vi "daq.io Embedded Machine Example Token.vi"(8 "error in":errorcluster) -> (0 "error out":errorcluster)   [LabVIEW 2013, in "daqio minimal.lvlib"]
doc: "This interactive example demonstrates how an NI Embedded device can used for continuous monitoring with daq.io. Tags and Events in this example are written on user demand but could also be triggered by monitored values. \n\nTo get started, <b>drag this example onto a Real-Time target in the Project Explorer, enter a valid Token in the block diagram</b> and run it interactively. You can also build an Executable and run it upon startup. To generate a Token, log in to your account on daq.io and go to your user page (click your user name next to logout button).\n\nThe NI System Configuration API is being used to monitor the status of the Embedded device. Please make sure its libraries are installed on the Embedded Device to get the best experience."
uses:
  daqio minimal.lvlib
  _typedefs/update-button.ctl
  _typedefs/trigger-button.ctl
  _typedefs/exmpl-states.ctl
  _typedefs/connection_FGV_commands.ctl
  _typedefs/daqio-reconnect-status.ctl
  _typedefs/daqio-Buffer-Commands.ctl
  <vilib>/nisyscfg/Close (System).vi
  _subs/daqio_Write_Multiple_single_Timestamp.vi
  <resource>/objmgr/nisysapi.rc
  <vilib>/nisyscfg/nisyscfg.lvlib
panel:
  out "Setpoint":dbl(slide) scale=0.0..150.0
  out "shutdown":bool
  out "Log":string[](array[string])
  in  "Stop":bool
  in  "Fire Event":T1
  in  "Select Event":u16(ring) items=["Safety Hood Status", "Manual Operation", "Shutting Down"]
  out "Time Stamp sent":timestamp
  in  "Event Data":string
  in  "Update Tags":T2
  out "connected":bool
  out "Speed (RPM)":dbl(knob) scale=0.0..2000.0
  out "Temperature Data":dbl(graph)
  out "RAM":dbl(slide) scale=0.0..100.0
  out "CPU":dbl(slide) scale=0.0..100.0
  in  "Value 3":string="1234-abc"
  in  "Value 2":string="XYZ 3000 Plus"
  in  "Tag 3":string="Serial Number"
  in  "Tag 2":string="Type"
  in  "Value 1":string="47.615459, -122.323804"
  in  "Tag 1":string="Location"
  out "Device Key":string
  # "Get your free account at daq.io first: sign up at daq.io."
  # "This Machine"
  # "(autogenerated in this example)"
  # "Please enter your \nToken in the block \ndiagram. Generate \nyour Token online."
  # "Device Tags"
  # "Use device tags to describe \nspecific parameters for each\ndevice. These can include the \nlocation, the serial number or\nother machine or location-\nspecific information. These\nfields are fully user-defined."
  # "Device Events"
  # "Use device events to signal\nany local event to daq.io. These\ncould include mechanical events\n(e.g. \"safety latch released\") or \nany change on the device that\nneeds to be tracked."
  # "Device Live Data Channels"
  # "Use device channels to transfer\ntime series data. All channels \nof the device will be visible in \nthe online data viewer. You \ncan build your own dashboard \nin the webbrowser and link it\nto exisiting channels."
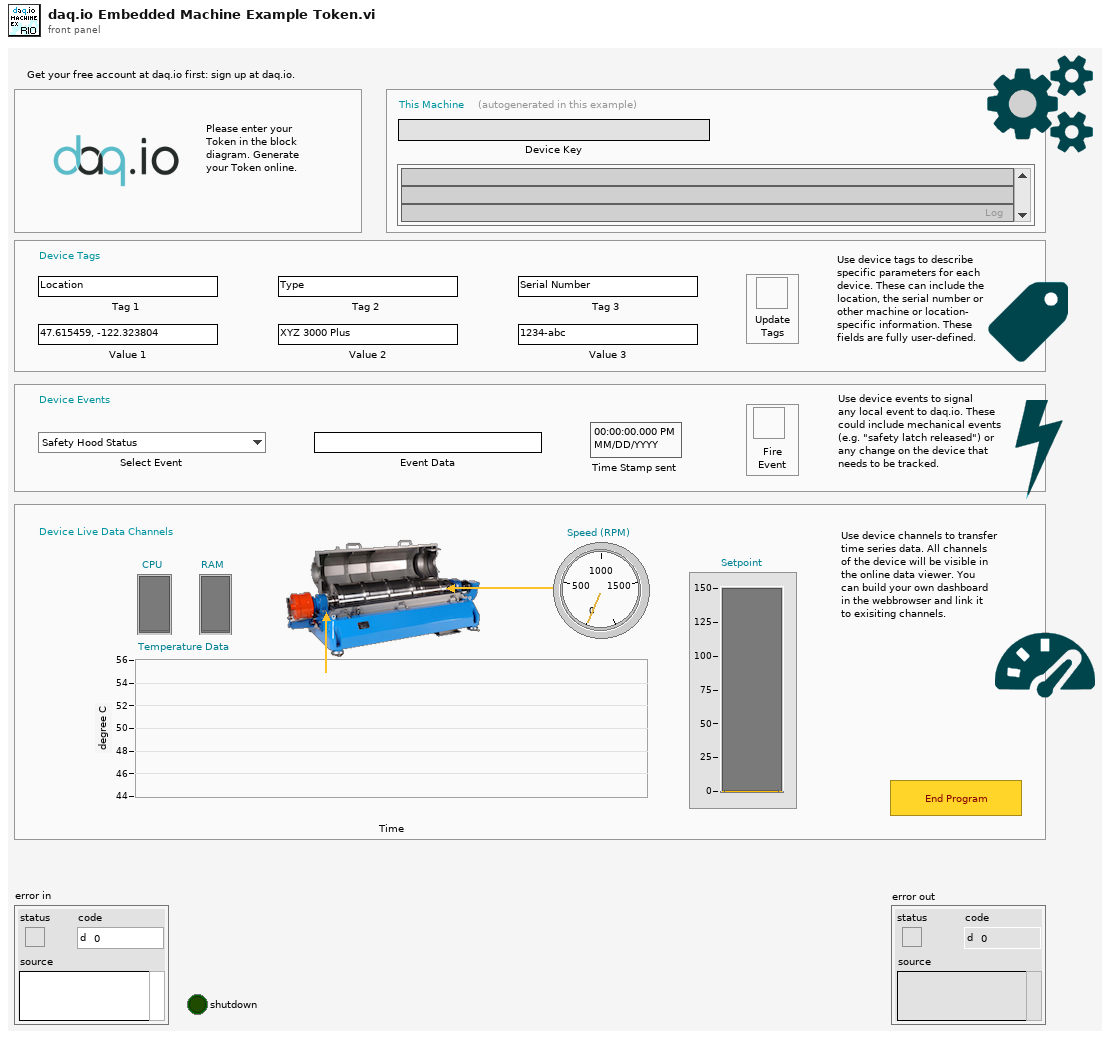
[diagram p1: front panel]
types:
  T1 = typedef "daqio minimal.lvlib/trigger-button.ctl" = bool
  T2 = typedef "daqio minimal.lvlib/update-button.ctl" = bool
  T3 = typedef "daqio minimal.lvlib/exmpl-states.ctl" = enum16{"idle", "time series", "fire events", "update tags", "end program", "create waveform", "create dashboard"}
  T4 = typedef "daqio minimal.lvlib/daqio-Type.ctl" = cluster{"daq.io ref":T5, "daq.io API Base":string, "Device Key":string, "Account ID":string, "online":bool, "SSL":bool}
  T5 = typedef "LabVIEWHTTPClient.lvlib/ClientHandle.ctl" = refnum<k1>
  T6 = typedef "daqio minimal.lvlib/connection_FGV_commands.ctl" = enum16{"Set Conn Stat", "Save Type", "Get Type from File", "Set Type", "Set Buffer", "Get"}
  T7 = typedef "daqio minimal.lvlib/daqio-reconnect-status.ctl" = enum16{"Reconnect success", "Reconnect failed", "Connected", "Offline"}
  T8 = typedef "daqio minimal.lvlib/daqio-Buffer-Commands.ctl" = enum16{"Add to Buffer", "Post from Buffer", "Clear Buffer", "Init"}
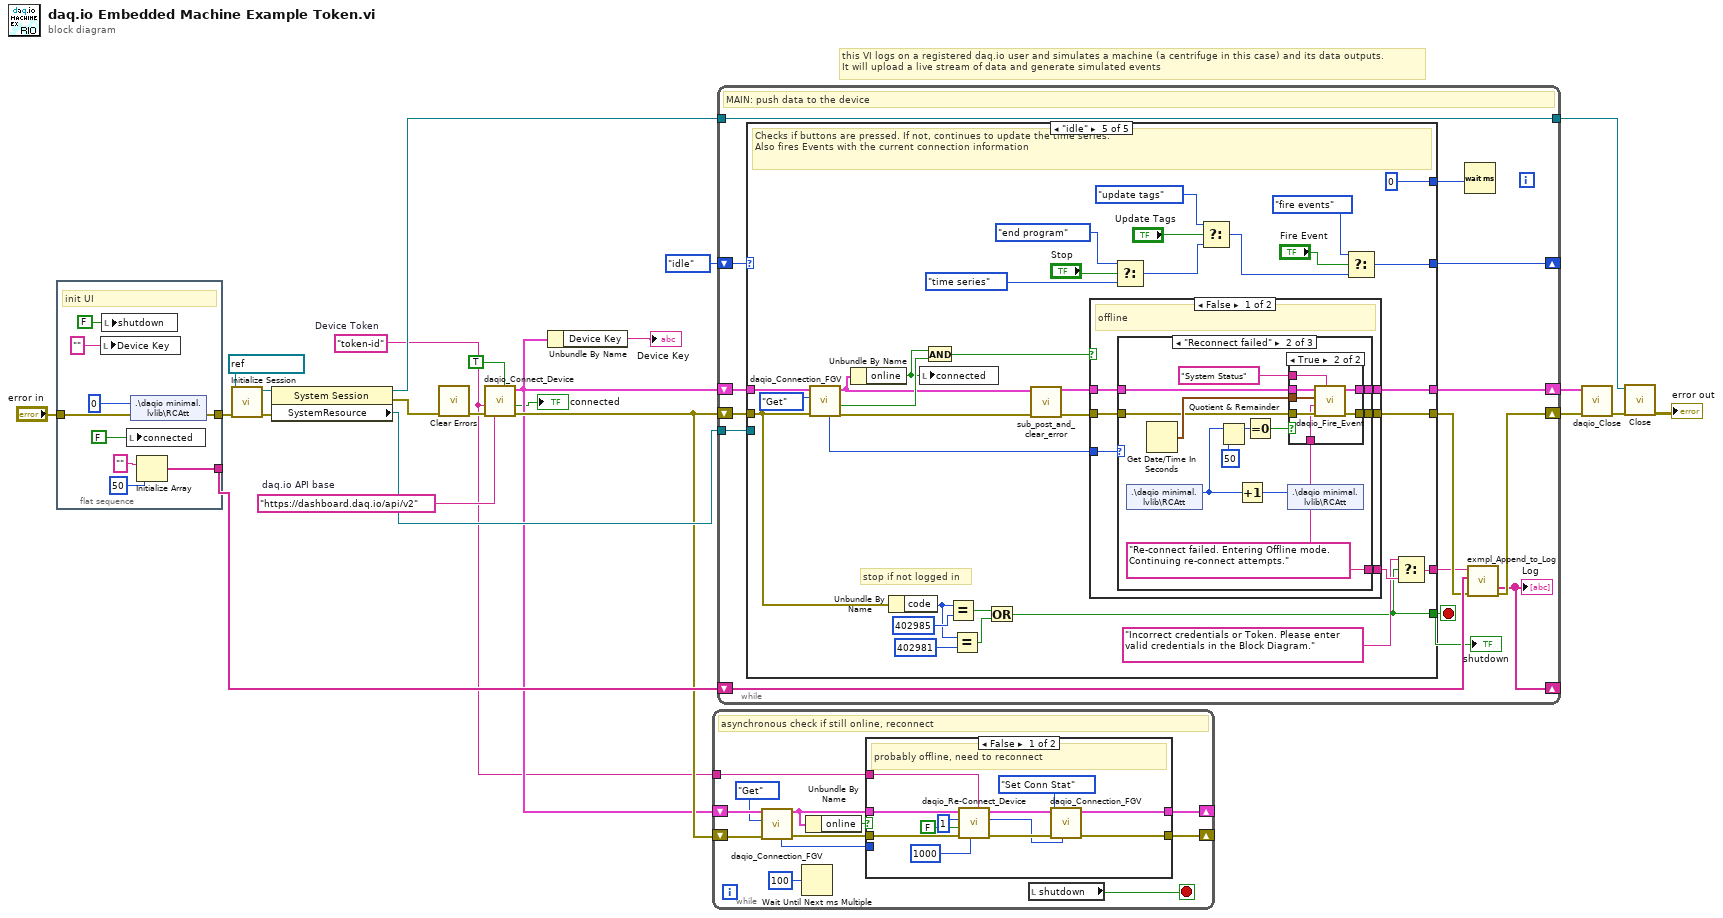
[diagram p0: block diagram]
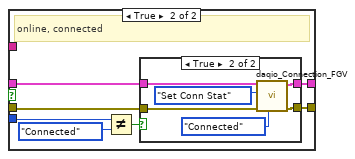
[diagram p2: hidden frame]
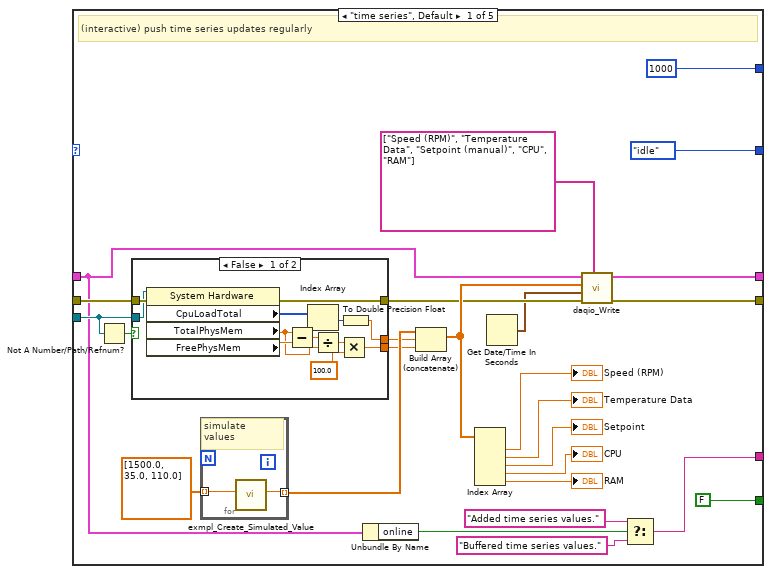
[diagram p4: hidden frame]
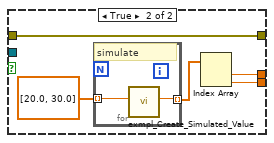
[diagram p5: hidden frame]
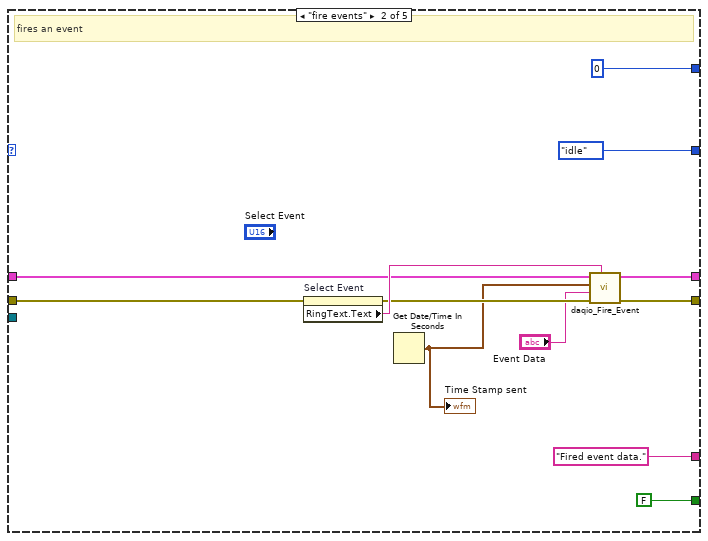
[diagram p6: hidden frame]
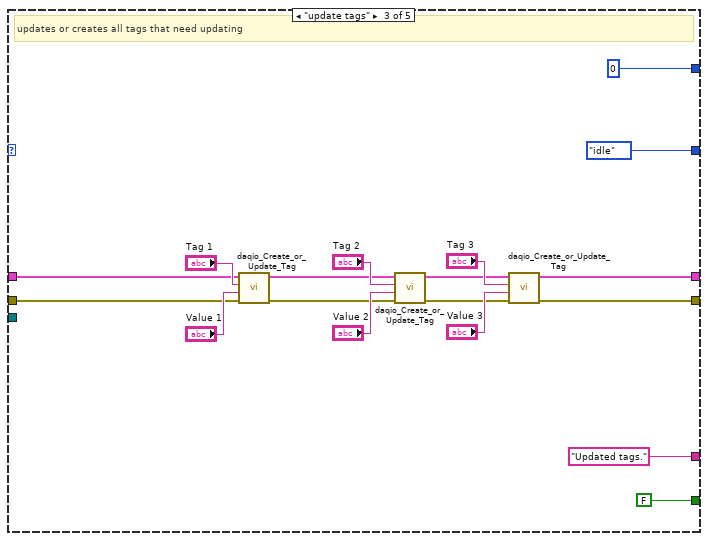
[diagram p7: hidden frame]
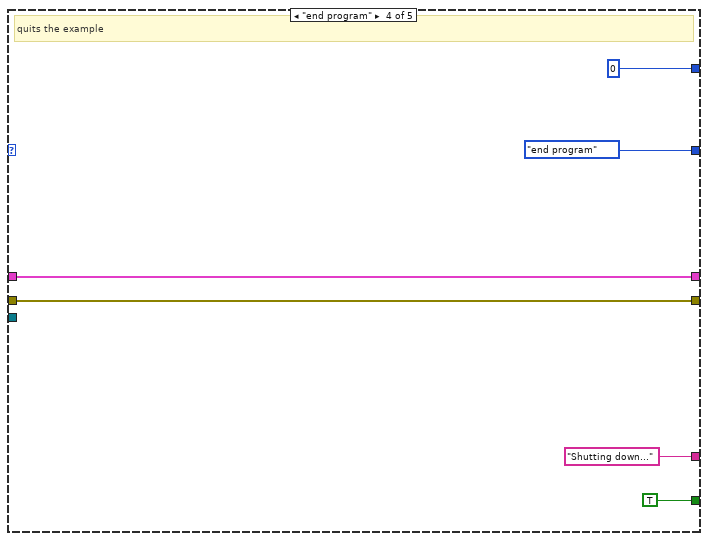
[diagram p8: hidden frame]
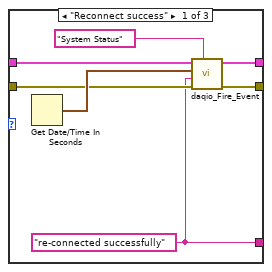
[diagram p9: hidden frame]
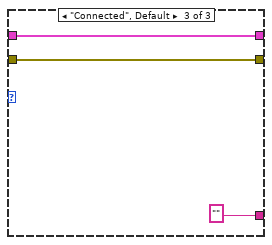
[diagram p11: hidden frame]
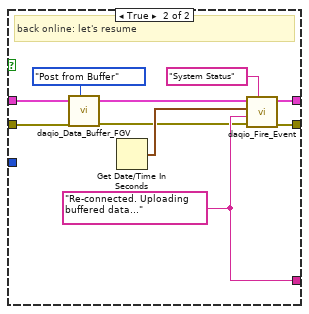
[diagram p12: hidden frame]
diagram:
  w1 = "token-id"  # Device Token
  w20 = "https://dashboard.daq.io/api/v2"  # daq.io API base
  # "this VI logs on a registered daq.io user and simulates a machine (a centrifuge in this case) and its data outputs. \nIt will upload a live stream of data and generate simulated events"
  n1 = flat-sequence {
    tunnel: [w26] -> w18
    tunnel: "error in" -> [w28]
    tunnel: [w29] -> w7
    frame #0 {
      # "init UI"
      n2 = local write "Device Key"("" ("log")) -> ()
      n3 = local write "shutdown"(FALSE ("shutdown")) -> ()
      n4 = local write "connected"(FALSE ("connected to daq.io")) -> ()
      n5 = shared-variable ".\\daqio minimal.lvlib\\RCAtt"(0 ("RCAtt"), error in=w28) -> (error out=w26:errorcluster)
      n6 = Initialize Array("" ("log"), 50 ("dimension size")) -> (w29:string[])
    }
  }
  n7 = call <vilib>:"Initialize Session.vi"("error in (no error)"=w18, "Target (localhost)"=refnum<k21> "localhost" ("Embedded Target (self)")) -> ("error out"=w12:errorcluster, "Session out"=w10:refnum<k21>)  [unwired: 8 in]
  n8 = property class="System Session"(reference=w10, error in=w12) -> (reference out=w9:refnum<k21>, error out=w11:errorcluster, "SystemResource"=w13:refnum<k20>)
  n9 = call <vilib>:"Clear Errors.vi"("error in (no error)"=w11) -> ("error out"=w4:errorcluster)  [unwired: 6 in]
  n10 = call "daqio_Connect_Device.vi"("Use SSL"=TRUE, "daq.io API base"=w20, "error in (no error)"=w4, "Device Token"=w1) -> ("error out"=w6:errorcluster, "connected successfully?"=→"connected":bool, "daq.io type out"=w5:T4)  [unwired: 5 in]
  n11 = Unbundle By Name(w5) -> ("Device Key"=→"Device Key":string)
  n12 = while {
    shift-right: [w37] -> _
    shift-left: w6 -> [w41]
    shift-right: [w38] -> _
    shift-left: w5 -> [w42]
    tunnel: w1 -> [w33]
    stop <- w44 stop-if-true
    # "asynchronous check if still online, reconnect"
    n13 = call "daqio_Connection_FGV.vi"("error in"=w41, "Enum"=connection_FGV_commands."Get", "daq.io type in"=w42) -> ("error out"=w39:errorcluster, "daq.io type out"=w35:T4, "Connection Status out"=w34:T7)  [unwired: 5 in, 1 out]
    n14 = Wait Until Next ms Multiple(millisecond multiple=u32 100) -> ()  [unwired: 1 out]
    n15 = Unbundle By Name(w35) -> ("online"=w36:bool)
    n16 = case shown="False" w36 {
      tunnel: w39 -> [w54 w58]
      tunnel: [w49 w61] -> w38
      tunnel: [w48 w60] -> w37
      tunnel: w35 -> [w47 w59]
      tunnel: w34 -> [_ w63]
      tunnel: w33 -> [w45 _]
      frame False {
        # "probably offline, need to reconnect"
        n17 = call "daqio_Re-Connect_Device.vi"("Token"=w45, "re-connect timeouts"=u32 1000, "error in"=w54, "override any errors"=FALSE, "re-connect attempts"=1, "daq.io type in"=w47) -> ("error out"=w53:errorcluster, "status"=w50:T7, "daq.io type out"=w52:T4)  [unwired: 3 in]
        n18 = call "daqio_Connection_FGV.vi"("Connection Status in"=w50, "error in"=w53, "Enum"=connection_FGV_commands."Set Conn Stat", "daq.io type in"=w52) -> ("error out"=w48:errorcluster, "daq.io type out"=w49:T4)  [unwired: 4 in, 2 out]
      }
      frame True {
        # "online, connected"
        n19 = Not Equal?(x=w63, y=daqio-reconnect-status."Connected") -> (x != y?=w57:bool)
        n20 = case shown="True" w57 {
          tunnel: [w65 w71] -> w61
          tunnel: [w64 w70] -> w60
          tunnel: w59 -> [w65 w69]
          tunnel: w58 -> [w64 w68]
          frame False {
          }
          frame True {
            n21 = call "daqio_Connection_FGV.vi"("Connection Status in"=daqio-reconnect-status."Connected", "error in"=w68, "Enum"=connection_FGV_commands."Set Conn Stat", "daq.io type in"=w69) -> ("error out"=w70:errorcluster, "daq.io type out"=w71:T4)  [unwired: 4 in, 2 out]
          }
        }
      }
    }
    n22 = local read "shutdown"() -> (w44:bool)
  }
  n23 = while {
    shift-right: [w77] -> w23
    shift-left: w6 -> [w74]
    shift-right: [w85] -> w21
    shift-left: w5 -> [w75]
    shift-right: [w83] -> _
    shift-left: exmpl-states."idle" -> [w84]
    tunnel: w13 -> [w81]
    tunnel: [w80] -> w15
    tunnel: w9 -> [w80]
    shift-right: [w76] -> _
    shift-left: w7 -> [w79]
    stop <- w72 stop-if-true
    # "MAIN: push data to the device"
    n24 = case shown="\"idle\"" w84 {
      tunnel: w75 -> [w86 w141 w152 w166 w180]
      tunnel: w74 -> [w104 w140 w151 w165 w179]
      tunnel: [w89 w138 w149 w166 w190] -> w85
      tunnel: [w88 w139 w150 w165 w189] -> w78
      tunnel: [exmpl-states."idle" exmpl-states."idle" exmpl-states."idle" exmpl-states."end program" w198] -> w83
      tunnel: [FALSE FALSE FALSE TRUE w174] -> w72
      tunnel: [u32 1000 ("milliseconds to wait") u32 0 ("milliseconds to wait") u32 0 ("milliseconds to wait") u32 0 ("milliseconds to wait") u32 0 ("milliseconds to wait")] -> w82
      tunnel: [w96 "Fired event data." ("log") "Updated tags." ("log") "Shutting down..." ("log") w183] -> w73
      tunnel: w81 -> [w102 _ _ _ _]
      frame "time series", Default {
        # "(interactive) push time series updates regularly"
        n25 = Not A Number/Path/Refnum?(number/path/refnum=w102) -> (NaN/Path/Refnum?=w101:bool)
        n26 = case shown="False" w101 {
          tunnel: w104 -> [w123 w124]
          tunnel: w102 -> [w122 _]
          tunnel: [w121 w124] -> w91
          tunnel: [w117 w125] -> w103
          tunnel: [w115 w126] -> w100
          frame False {
            n27 = property class="System Hardware"(reference=w122, error in=w123) -> (error out=w121:errorcluster, "CpuLoadTotal"=w120:u32[], "TotalPhysMem"=w112:dbl, "FreePhysMem"=w113:dbl)  [unwired: 1 out]
            n28 = Subtract(x=w112, y=w113) -> (x-y=w114:dbl)
            n29 = Index Array(array=w120) -> (element=w116:u32)  [unwired: 1 in]
            n30 = Divide(x=w114, y=w112) -> (x/y=w119:dbl)
            n31 = Multiply(x=w119, y=100.0) -> (x*y=w117:dbl)
            n32 = To Double Precision Float(number=w116) -> (double precision float=w115:dbl)
          }
          frame True {
            n33 = for {
              tunnel: [w130] -> w127 mode=indexing
              tunnel: dbl[] [20.0, 30.0] -> [w129] mode=indexing
              # "simulate"
              n34 = call "exmpl_Create_Simulated_Value.vi"("offset"=w129) -> ("Numeric"=w130:dbl)  [unwired: 9 in, 1 out]
            }
            n35 = Index Array(array=w127) -> (element #1=w126:dbl, element #2=w125:dbl)  [unwired: 2 in]
          }
        }
        n36 = for {
          tunnel: [w132] -> w111 mode=indexing
          tunnel: dbl[] [1500.0, 35.0, 110.0] -> [w131] mode=indexing
          # "simulate\nvalues"
          n37 = call "exmpl_Create_Simulated_Value.vi"("offset"=w131) -> ("Numeric"=w132:dbl)  [unwired: 9 in, 1 out]
        }
        n38 = Unbundle By Name(w86) -> ("online"=w99:bool)
        n39 = Build Array (concatenate)(w111, w100, w103) -> (w92:dbl[])
        n40 = Index Array(array=w92) -> (element #1=→"Speed (RPM)":dbl, element #2=→"Temperature Data":dbl, element #3=→"Setpoint":dbl, element #4=→"CPU":dbl, element #5=→"RAM":dbl)  [unwired: 5 in]
        n41 = Get Date/Time In Seconds() -> (seconds since 1Jan1904=w87:timestamp)
        n42 = call-poly "daqio_Write.vi"("daq.io Device Channel Keys"=string[] ["Speed (RPM)", "Temperature Data", "Setpoint (manual)", "CPU", "RAM"], "error in (no error)"=w91, "Timestamp"=w87, "Values"=w92, "daq.io type in"=w86) -> ("error out"=w88:errorcluster, "daq.io type out"=w89:T4)  [unwired: 5 in]
        n43 = Select(t="Added time series values." ("log"), s=w99, f="Buffered time series values." ("log")) -> (s? t:f=w96:string)
      }
      frame "fire events" {
        # "fires an event"
        n44 = property on="Select Event" class="Ring (strict)"(error in=w140) -> (error out=w143:errorcluster, "RingText.Text"=w144:string)  [unwired: 1 in, 1 out]
        n45 = Get Date/Time In Seconds() -> (seconds since 1Jan1904=w133:timestamp)
        "Time Stamp sent" <- w133
        n46 = call "daqio_Fire_Event.vi"("Event Key"=w144, "error in (no error)"=w143, "Event Value"="Event Data", "Event Date and Time"=w133, "daq.io type in"=w141) -> ("error out"=w139:errorcluster, "daq.io type out"=w138:T4)  [unwired: 5 in]
      }
      frame "update tags" {
        # "updates or creates all tags that need updating"
        n47 = call "daqio_Create_or_Update_Tag.vi"("error in (no error)"=w151, "Tag Value"="Value 1", "Tag Key"="Tag 1", "daq.io type in"=w152) -> ("error out"=w156:errorcluster, "daq.io type out"=w153:T4)  [unwired: 5 in, 1 out]
        n48 = call "daqio_Create_or_Update_Tag.vi"("error in (no error)"=w156, "Tag Value"="Value 2", "Tag Key"="Tag 2", "daq.io type in"=w153) -> ("error out"=w155:errorcluster, "daq.io type out"=w154:T4)  [unwired: 5 in, 1 out]
        n49 = call "daqio_Create_or_Update_Tag.vi"("error in (no error)"=w155, "Tag Value"="Value 3", "Tag Key"="Tag 3", "daq.io type in"=w154) -> ("error out"=w150:errorcluster, "daq.io type out"=w149:T4)  [unwired: 5 in, 1 out]
      }
      frame "end program" {
        # "quits the example"
      }
      frame "idle" {
        # "stop if not logged in"
        # "Checks if buttons are pressed. If not, continues to update the time series. \nAlso fires Events with the current connection information"
        n50 = call "daqio_Connection_FGV.vi"("error in"=w179, "Enum"=connection_FGV_commands."Get", "daq.io type in"=w180) -> ("error out"=w175:errorcluster, "Buffered Data exists?"=w187:bool, "daq.io type out"=w178:T4, "Connection Status out"=w185:T7)  [unwired: 5 in]
        n51 = Unbundle By Name(w178) -> ("online"=w186:bool)
        n52 = Unbundle By Name(w179) -> ("code"=w171:i32)
        n53 = local write "connected"(w186) -> ()
        n54 = And(x=w186, y=w187) -> (x .and. y?=w188:bool)
        n55 = Equal?(x=w171, y=402985) -> (x = y?=w173:bool)
        n56 = Equal?(x=w171, y=402981) -> (x = y?=w169:bool)
        n57 = Or(x=w173, y=w169) -> (x .or. y?=w174:bool)
        n58 = call "sub_post_and_clear_error.vi"("error in (no error)"=w175, "daq.io type in"=w178) -> ("error out"=w176:errorcluster, "daq.io type out"=w177:T4)  [unwired: 8 in]
        n59 = case shown="False" w188 {
          tunnel: w177 -> [w203 w247]
          tunnel: w176 -> [w204 w246]
          tunnel: [w207 w244] -> w184
          tunnel: [w206 w240] -> w190
          tunnel: [w205 w239] -> w189
          tunnel: w185 -> [w202 _]
          frame False {
            # "offline"
            n60 = case shown="\"Reconnect failed\"" w202 {
              tunnel: [w208 w220 ""] -> w207
              tunnel: [w212 w221 w237] -> w206
              tunnel: [w211 w222 w236] -> w205
              tunnel: w204 -> [w210 w224 w236]
              tunnel: w203 -> [w209 w223 w237]
              frame "Reconnect success" {
                w208 = "re-connected successfully"
                n61 = Get Date/Time In Seconds() -> (seconds since 1Jan1904=w214:timestamp)
                n62 = call "daqio_Fire_Event.vi"("Event Key"="System Status", "error in (no error)"=w210, "Event Value"=w208, "Event Date and Time"=w214, "daq.io type in"=w209) -> ("error out"=w211:errorcluster, "daq.io type out"=w212:T4)  [unwired: 5 in]
              }
              frame "Reconnect failed" {
                w220 = "Re-connect failed. Entering Offline mode. Continuing re-connect attempts."
                n63 = shared-variable ".\\daqio minimal.lvlib\\RCAtt"() -> (w216:i32)  [unwired: 1 in, 1 out]
                n64 = Get Date/Time In Seconds() -> (seconds since 1Jan1904=w226:timestamp)
                n65 = Quotient & Remainder(x=w216, y=50) -> (x-y*floor(x/y)=w219:i32)  [unwired: 1 out]
                n66 = Increment(x=w216) -> (x+1=w215:i32)
                n67 = Equal To 0?(x=w219) -> (x = 0?=w218:bool)
                n68 = shared-variable ".\\daqio minimal.lvlib\\RCAtt"(w215) -> ()  [unwired: 1 in, 1 out]
                n69 = case shown="True" w218 {
                  tunnel: w226 -> [_ w235]
                  tunnel: "System Status" ("Event Key") -> [_ w234]
                  tunnel: w224 -> [w227 w233]
                  tunnel: w223 -> [w228 w232]
                  tunnel: [w227 w231] -> w222
                  tunnel: [w228 w230] -> w221
                  tunnel: w220 -> [_ w229]
                  frame False {
                  }
                  frame True {
                    n70 = call "daqio_Fire_Event.vi"("Event Key"=w234, "error in (no error)"=w233, "Event Value"=w229, "Event Date and Time"=w235, "daq.io type in"=w232) -> ("error out"=w231:errorcluster, "daq.io type out"=w230:T4)  [unwired: 5 in]
                  }
                }
              }
              frame "Connected", Default {
              }
            }
          }
          frame True {
            w244 = "Re-connected. Uploading buffered data..."
            # "back online: let's resume"
            n71 = call "daqio_Data_Buffer_FGV.vi"("Buffer Command"=daqio-Buffer-Commands."Post from Buffer", "error in (no error)"=w246, "daq.io type in"=w247) -> ("error out"=w242:errorcluster, "daq.io type out"=w243:T4)  [unwired: 7 in]
            n72 = Get Date/Time In Seconds() -> (seconds since 1Jan1904=w245:timestamp)
            n73 = call "daqio_Fire_Event.vi"("Event Key"="System Status", "error in (no error)"=w242, "Event Value"=w244, "Event Date and Time"=w245, "daq.io type in"=w243) -> ("error out"=w239:errorcluster, "daq.io type out"=w240:T4)  [unwired: 5 in]
          }
        }
        n74 = Select(t=exmpl-states."end program", s="Stop", f=exmpl-states."time series") -> (s? t:f=w193:T3)
        n75 = Select(t=exmpl-states."update tags", s="Update Tags", f=w193) -> (s? t:f=w199:T3)
        n76 = Select(t=exmpl-states."fire events", s="Fire Event", f=w199) -> (s? t:f=w198:T3)
        n77 = Select(t="Incorrect credentials or Token. Please enter valid credentials in the Block Diagram.", s=w174, f=w184) -> (s? t:f=w183:string)
      }
    }
    "shutdown" <- w72
    n78 = Wait (ms)(milliseconds to wait=w82) -> ()  [unwired: 1 out]
    n79 = call "exmpl_Append_to_Log.vi"("error in (no error)"=w78, "Log Array in"=w79, "Log Message"=w73) -> ("error out"=w77:errorcluster, "Log Array out"=w76:string[])  [unwired: 7 in]
    "Log" <- w76
  }
  n80 = call "daqio_Close.vi"("error in (no error)"=w23, "daq.io type"=w21) -> ("error out"=w17:errorcluster)  [unwired: 9 in]
  n81 = call-poly <vilib>:"Close.vi"("error in (no error)"=w17, "Session in"=w15) -> ("error out"=→"error out":errorcluster)  [unwired: 9 in]
